vi "testInternalMemorySwap.vi"(8 "error in (no error)":errorcluster, 11 "TestCase in":refnum<class "Memory Manager Unit Tests.lvclass">) -> (0 "error out":errorcluster, 3 "TestCase out":refnum<class "Memory Manager Unit Tests.lvclass">)   [LabVIEW 2016, in "Memory Manager Unit Tests.lvclass"]
uses:
  Memory Manager Unit Tests.lvclass
  Library/Classes/Pointer/Memory.Pointer.lvclass/Memory.Pointer.ctl
  Library/Classes/Pointer.Internal/Methods/Memory.Pointer.Internal.Swap.Safe.vi
  Library/Classes/Pointer/Methods/Memory.Pointer.Read.Safe.1D.U8.vi
  Library/Classes/Pointer/Accessors/Get Size.vi
  Library/Classes/Pointer.Internal/Methods/Memory.Pointer.Internal.Swap.Unsafe.vi
  Library/Classes/Pointer/Methods/Memory.Pointer.Read.Unsafe.1D.U8.vi
  Library/Classes/Pointer/Methods/Memory.Pointer.Parameter Check.Size.1D (Power of 2).vi
  Library/Classes/Pointer/Accessors/Get Address.vi
  Library/Classes/Pointer/Accessors/Set Address.vi
  Library/Classes/Pointer/Methods/Memory.Pointer.Errors.vi
  Library/Classes/Pointer/Methods/Memory.Pointer.Errors.Buffer Underflow.vi
  Library/Classes/Pointer/Methods/Memory.Pointer.Parameter Check.Size.0D.vi
  Library/Classes/Pointer/Methods/Memory.Pointer.Errors.Create Error.vi
  Submodules/Static Error Handling/Source/Library/VIs/Static Error Handling.Source Buffer.Write.String.vi
  Submodules/Static Error Handling/Source/Library/VIs/Static Error Handling.Source Buffer.Write.Numeric.Scalar.Base10.vi
  Submodules/Static Error Handling/Source/Library/VIs/Static Error Handling.Source Buffer.Write.Numeric.Scalar.Base10 (U64).vi
  Library/Classes/Pointer/Methods/Memory.Pointer.Errors.Out of Bounds.vi
  Submodules/Static Error Handling/Source/Library/VIs/Static Error Handling.Error Cluster Constant.vi
  Submodules/Static Error Handling/Source/Library/VIs/Static Error Handling.Error Cluster Constant (256B).vi
  Submodules/Static Error Handling/Source/Library/VIs/Static Error Handling.Parameters.Status.Set.vi
  Submodules/Static Error Handling/Source/Library/VIs/Static Error Handling.Parameters.Code.Set.vi
  Submodules/Static Error Handling/Source/Library/VIs/Static Error Handling.Parameters.VI Source.Set.vi
  Library/Constants/Memory.Constants.vi
  Library/Constants/Memory.Constants.Library Name.vi
  Library/Classes/Pointer/Methods/Memory.Pointer.Errors.Get Info.vi
  Library/Classes/Pointer/Methods/Memory.Pointer.Errors.Write Pointer Size.vi
  Library/Classes/Pointer.Internal/Memory.Pointer.Internal.lvclass
  C:/Git/Personal/LabVIEW-Memory-Manager/Source/Library/Classes/Pointer/Memory.Pointer.lvclass
  <vilib>/addons/_JKI Toolkits/VI Tester/TestCase.llb/TestCase.lvclass
  Library/Classes/Pointer/Memory.Pointer.lvclass
  C:/Program Files (x86)/National Instruments/LabVIEW 2016/vi.lib/addons/_JKI Toolkits/VI Tester/TestCase.llb/TestCase.lvclass
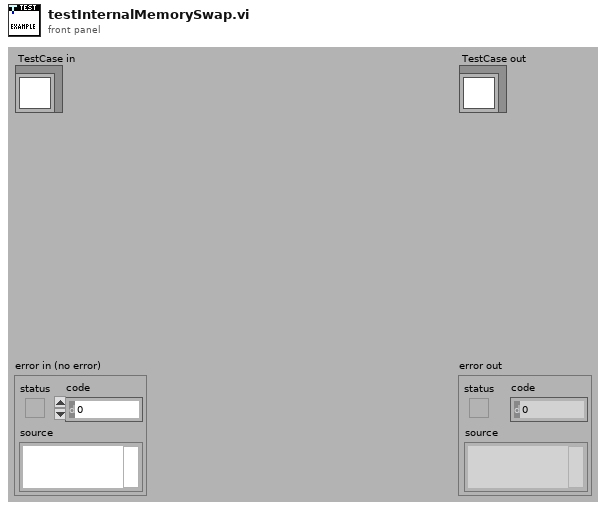
[diagram p1: front panel]
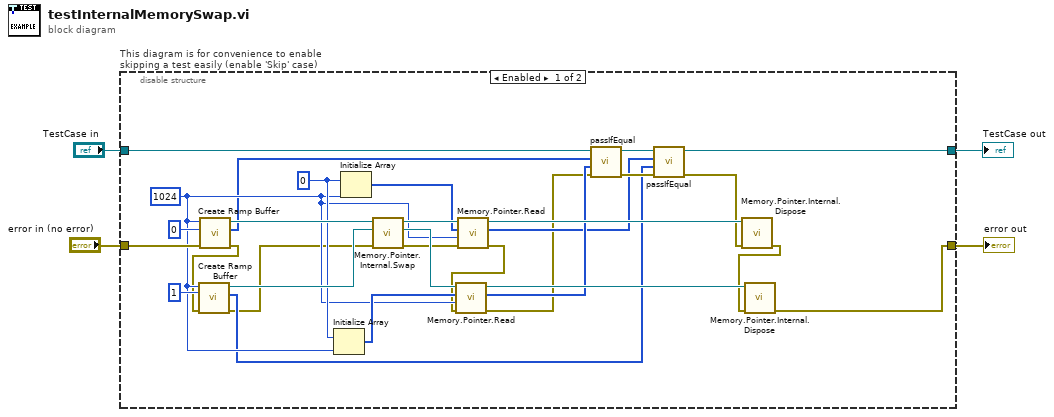
[diagram p0: block diagram]
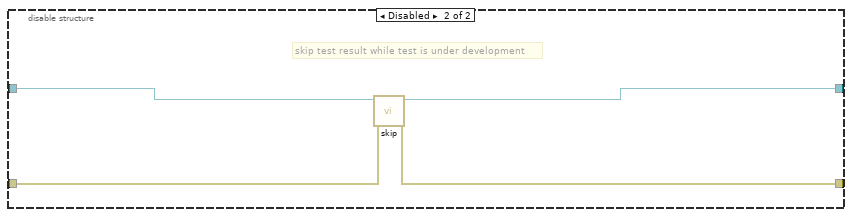
[diagram p2: hidden frame]
diagram:
  n1 = disable-structure "This diagram is for convenience to enable skipping a test easily (enable 'Skip' case)" shown="Enabled" {
    disable-tunnel: "TestCase in" -> [w33 w37]
    disable-tunnel: [w14 w35] -> w1
    disable-tunnel: [w10 w36] -> w3
    disable-tunnel: "error in (no error)" -> [w25 w34]
    frame Enabled {
      w23 = u8 0 ("Initial Value")
      w21 = u64 1024 ("Size")
      n2 = call "Create Ramp Buffer.vi"("error in (no error)"=w25, "initial value"=u8 0 ("Initial Value"), "size"=w21) -> ("error out"=w6:errorcluster, "buffer out"=w18:u8[], "pointer out"=w30:refnum<class "Memory.Pointer.Internal.lvclass">)  [unwired: 6 in]
      n3 = call "Create Ramp Buffer.vi"("error in (no error)"=w6, "initial value"=u8 1 ("Initial Value"), "size"=w21) -> ("error out"=w5:errorcluster, "buffer out"=w13:u8[], "pointer out"=w29:refnum<class "Memory.Pointer.Internal.lvclass">)  [unwired: 6 in]
      n4 = Initialize Array(w23, w21) -> (w24:u8[])
      n5 = Initialize Array(w23, w21) -> (w22:u8[])
      n6 = call-poly "Memory.Pointer.Internal.Swap.vi"("error in (no error)"=w5, "pointer b"=w29, "pointer a"=w30) -> ("error out"=w26:errorcluster, "pointer b"=w28:refnum<class "Memory.Pointer.Internal.lvclass">, "pointer a"=w27:refnum<class "Memory.Pointer.Internal.lvclass">)  [unwired: 6 in]
      n7 = call-poly "Memory.Pointer.Read.vi"("error in (no error)"=w26, "count"=w21, "buffer in"=w22, "pointer in"=w27) -> ("error out"=w8:errorcluster, "buffer out"=w12:u8[], "pointer out"=w19:refnum<class "Memory.Pointer.Internal.lvclass">)  [unwired: 4 in, 1 out]
      n8 = call-poly "Memory.Pointer.Read.vi"("error in (no error)"=w8, "count"=w21, "buffer in"=w24, "pointer in"=w28) -> ("error out"=w7:errorcluster, "buffer out"=w17:u8[], "pointer out"=w20:refnum<class "Memory.Pointer.Internal.lvclass">)  [unwired: 4 in, 1 out]
      n9 = call-dynamic "passIfEqual.vi"("error in (no error)"=w7, "y"=w17, "x"=w18, "TestCase in"=w33) -> ("error out"=w16:errorcluster, "TestCase out"=w15:refnum<class "Memory Manager Unit Tests.lvclass">)  [unwired: 6 in]
      n10 = call-dynamic "passIfEqual.vi"("error in (no error)"=w16, "y"=w13, "x"=w12, "TestCase in"=w15) -> ("error out"=w11:errorcluster, "TestCase out"=w14:refnum<class "Memory Manager Unit Tests.lvclass">)  [unwired: 6 in]
      n11 = call "Memory.Pointer.Internal.Dispose.vi"("error in (no error)"=w11, "pointer"=w19) -> ("error out"=w9:errorcluster)  [unwired: 9 in]
      n12 = call "Memory.Pointer.Internal.Dispose.vi"("error in (no error)"=w9, "pointer"=w20) -> ("error out"=w10:errorcluster)  [unwired: 9 in]
    }
    frame Disabled {
      # "skip test result while test is under development"
      n13 = call <vilib>:"skip.vi"("error in (no error)"=w34, "TestCase in"=w37) -> ("error out"=w36:errorcluster, "TestCase out"=w35:refnum<class "Memory Manager Unit Tests.lvclass">)  [unwired: 8 in]
    }
  }
  "error out" <- w3
  "TestCase out" <- w1
